vi "StopProcesses.vi"(8 "error in (no error)":errorcluster, 9 "timeout in ms (-1)":i32=-1, 11 "SMO":refnum<class "SMO.lvclass">) -> (0 "error out":errorcluster, 3 "SMO out":refnum<class "SMO.lvclass">)   [LabVIEW 2013, in "SMO.lvclass"]
doc: "Stops all processes in the JKI SMO.\n\n---------------------------------------------------------------\nJKI State Machine Objects™\nhttp://jki.net/state-machine-objects/\nCopyright (C) 2005-2015, JKI <info@jki.net>\nALL RIGHTS RESERVED"
uses:
  SMO.lvclass
panel:
  # "For instructions on how to use the JKI State Machine Objects, examples and video tutorials, visit:\nhttp://jki.net/state-machine-objects/\n\nJKI State Machine Objects™\nhttp://jki.net/state-machine-objects/\nCopyright (C) 2005-2015, JKI <info@jki.net>\nALL RIGHTS RESERVED"
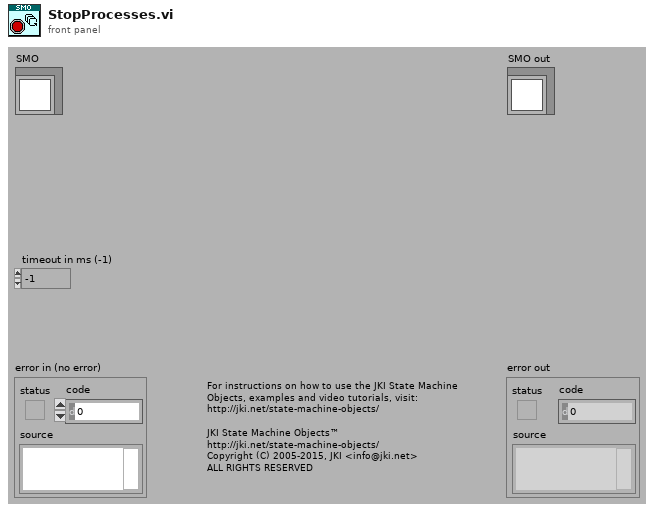
[diagram p1: front panel]
types:
  T1 = typedef "SMO.lvclass/Process Error Notification--Cluster.ctl" = cluster{"error":errorcluster}
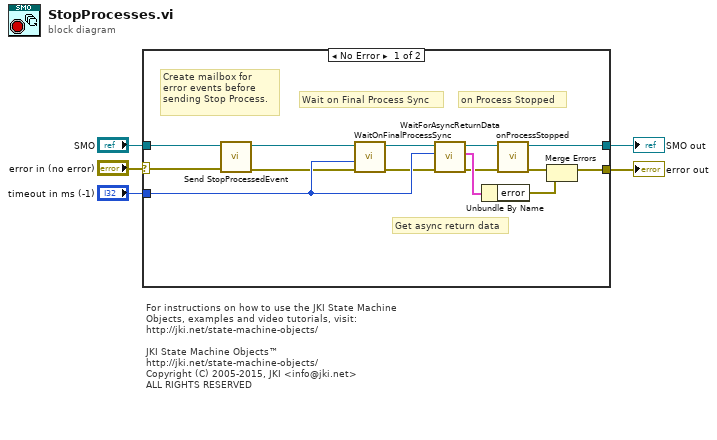
[diagram p0: block diagram]
diagram:
  # "For instructions on how to use the JKI State Machine Objects, examples and video tutorials, visit:\nhttp://jki.net/state-machine-objects/\n\nJKI State Machine Objects™\nhttp://jki.net/state-machine-objects/\nCopyright (C) 2005-2015, JKI <info@jki.net>\nALL RIGHTS RESERVED"
  n1 = case shown="No Error" "error in (no error)" {
    selector: "error in (no error)" -> [w15 w21]
    tunnel: [w7 w21] -> w1
    tunnel: [w10 w20] -> w3
    tunnel: "SMO" -> [w16 w20]
    tunnel: "timeout in ms (-1)" -> [w19 _]
    frame No Error {
      # "on Process Stopped"
      # "Get async return data"
      # "Wait on Final Process Sync"
      # "Create mailbox for\nerror events before\nsending Stop Process."
      n2 = call "Send StopProcessedEvent.vi"("error in (no error)"=w15, "SMO"=w16) -> ("error out"=w17:errorcluster, "SMO out"=w18:refnum<class "SMO.lvclass">)  [unwired: 8 in]
      n3 = call "WaitOnFinalProcessSync.vi"("error in (no error)"=w17, "timeout in ms (-1)"=w19, "SMO"=w18) -> ("error out"=w13:errorcluster, "SMO out"=w14:refnum<class "SMO.lvclass">)  [unwired: 7 in]
      n4 = call "WaitForAsyncReturnData.vi"("error in (no error)"=w13, "timeout in ms (-1)"=w19, "SMO"=w14) -> ("error out"=w9:errorcluster, "Process Notification"=w12:T1, "SMO out"=w11:refnum<class "SMO.lvclass">)  [unwired: 6 in]
      n5 = Unbundle By Name(w12) -> ("error"=w6:errorcluster)
      n6 = call-dynamic "onProcessStopped.vi"("error in (no error)"=w9, "SMO"=w11) -> ("error out"=w8:errorcluster, "SMO out"=w10:refnum<class "SMO.lvclass">)  [unwired: 8 in]
      n7 = Merge Errors(w8, w6) -> (w7:errorcluster)
    }
    frame Error {
    }
  }
  "error out" <- w1
  "SMO out" <- w3
